vi "Adjust Splitter.vi"(8 "error in (no error)":errorcluster caption="错误输入（无错误）", 11 "PanelRootNode 输入":refnum<class "PanelRootNode.lvclass"> caption="DNL_LabVIEW Object in") -> (0 "error out":errorcluster caption="错误输出", 3 "PanelRootNode 输出":refnum<class "PanelRootNode.lvclass"> caption="DNL_LabVIEW Object out")   [LabVIEW 2016, in "PanelRootNode.lvclass"]
uses:
  PanelRootNode.lvclass
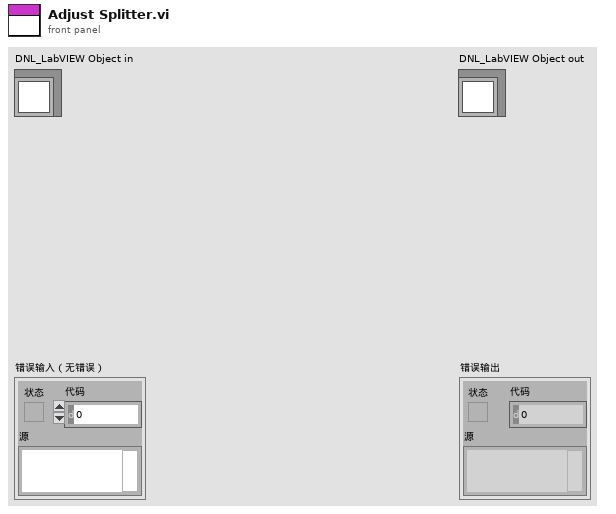
[diagram p1: front panel]
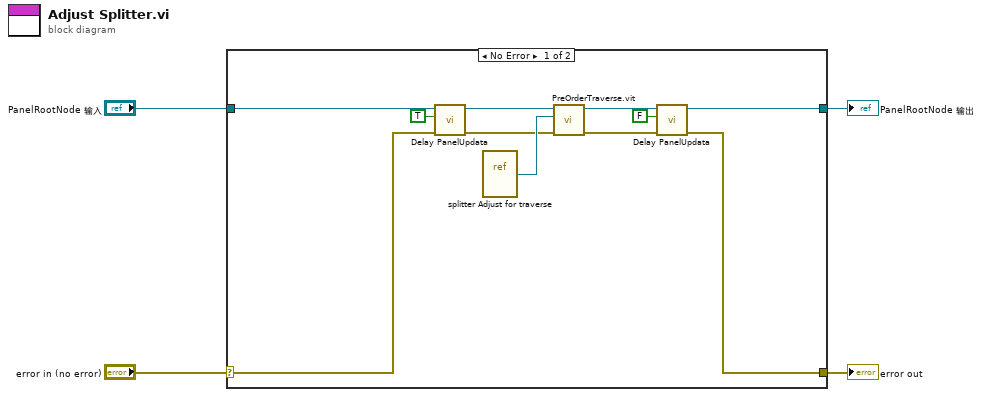
[diagram p0: block diagram]
diagram:
  n1 = case shown="No Error" "error in (no error)" {
    selector: "error in (no error)" -> [w9 w17]
    tunnel: [w7 w17] -> w3
    tunnel: [w11 w16] -> w1
    tunnel: "PanelRootNode 输入" -> [w14 w16]
    frame No Error {
      n2 = call "Delay PanelUpdata.vi"("error in"=w9, "延迟前面板更新"=TRUE, "PanelRootNode 输入"=w14) -> ("error out"=w10:errorcluster, "PanelRootNode 输出"=w13:refnum<class "PanelRootNode.lvclass">)  [unwired: 7 in]
      n3 = vi-ref "splitter Adjust for traverse.vi"() -> (w15:refnum<vi>)
      n4 = call-dynamic "PreOrderTraverse.vit"("error in"=w10, "vi reference"=w15, "PanelLinkNode 输入"=w13) -> ("error out"=w8:errorcluster, "PanelLinkNode 输出"=w12:refnum<class "PanelRootNode.lvclass">)  [unwired: 5 in, 2 out]
      n5 = call "Delay PanelUpdata.vi"("error in"=w8, "延迟前面板更新"=FALSE, "PanelRootNode 输入"=w12) -> ("error out"=w7:errorcluster, "PanelRootNode 输出"=w11:refnum<class "PanelRootNode.lvclass">)  [unwired: 7 in]
    }
    frame Error {
    }
  }
  "error out" <- w3
  "PanelRootNode 输出" <- w1
